vi "Check mouse in some control area.vi"(10 "Total Bounds Rect":T2, 11 "Coords":T1) -> (2 "In the Control?":bool)   [LabVIEW 2021]
doc: "check mouse is in the control area, when mouse click.\n2014-11-14 12:30:35\n蒋松\njiangsong@outlook.com"
uses:
  <vilib>/Utility/miscctls.llb/LVRectTypeDef.ctl
  <vilib>/Utility/miscctls.llb/LVPoint32TypeDef.ctl
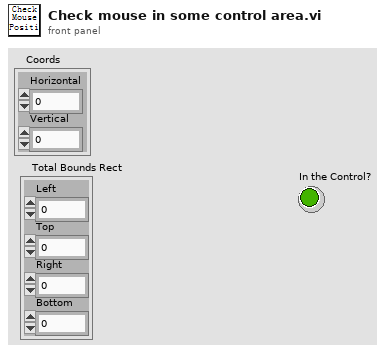
[diagram p1: front panel]
types:
  T1 = typedef "LVPoint32TypeDef.ctl" = cluster{"Horizontal":i32, "Vertical":i32}
  T2 = typedef "LVRectTypeDef.ctl" = cluster{"Left":i16, "Top":i16, "Right":i16, "Bottom":i16}
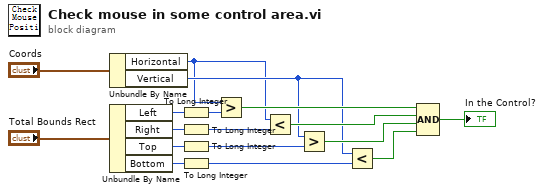
[diagram p0: block diagram]
diagram:
  n1 = Unbundle By Name("Coords") -> ("Horizontal"=w9:i32, "Vertical"=w12:i32)
  n2 = Unbundle By Name("Total Bounds Rect") -> ("Left"=w8:i16, "Right"=w11:i16, "Top"=w10:i16, "Bottom"=w13:i16)
  n3 = To Long Integer(number=w8) -> (32bit integer=w5:i32)
  n4 = To Long Integer(number=w11) -> (32bit integer=w3:i32)
  n5 = To Long Integer(number=w10) -> (32bit integer=w2:i32)
  n6 = To Long Integer(number=w13) -> (32bit integer=w4:i32)
  n7 = Greater?(x=w9, y=w5) -> (0:w14:bool)
  n8 = Less?(x=w9, y=w3) -> (x < y?=w15:bool)
  n9 = Greater?(x=w12, y=w2) -> (0:w16:bool)
  n10 = Less?(x=w12, y=w4) -> (x < y?=w17:bool)
  n11 = Compound Arithmetic op=AND(w14, w15, w16, w17) -> (→"In the Control?":bool)
